vi "insert_block.vi"(8 "direction":enum16{"up", "right", "down", "left"}(ring), 9 "block_type":T1(ring), 10 "position":cluster{"x":u8, "y":u8}, 11 "plate arr":u8[][](array[numeric])) -> (0 "valid?":bool, 3 "return plate":u8[][](array[numeric]))   [LabVIEW 2024]
uses:
  <vilib>/Analysis/coordinate.llb/2D Cartesian Coordinate Rotation (Array).vi
  <vilib>/Analysis/coordinate.llb/2D Cartesian Coordinate Rotation (Scalar).vi
  <vilib>/Analysis/NI_AALPro.lvlib
panel:
  out "熬簿":cluster{"x out":dbl, "y out":dbl}
  # "const table for plaing blocks"
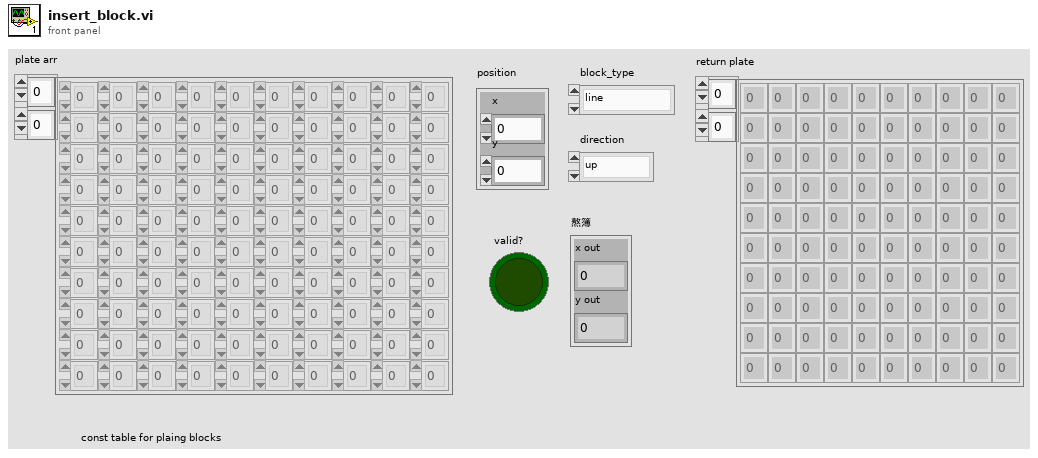
[diagram p1: front panel]
types:
  T1 = enum16{"line", "block", "T", "L", "rev_L", "undefined"}
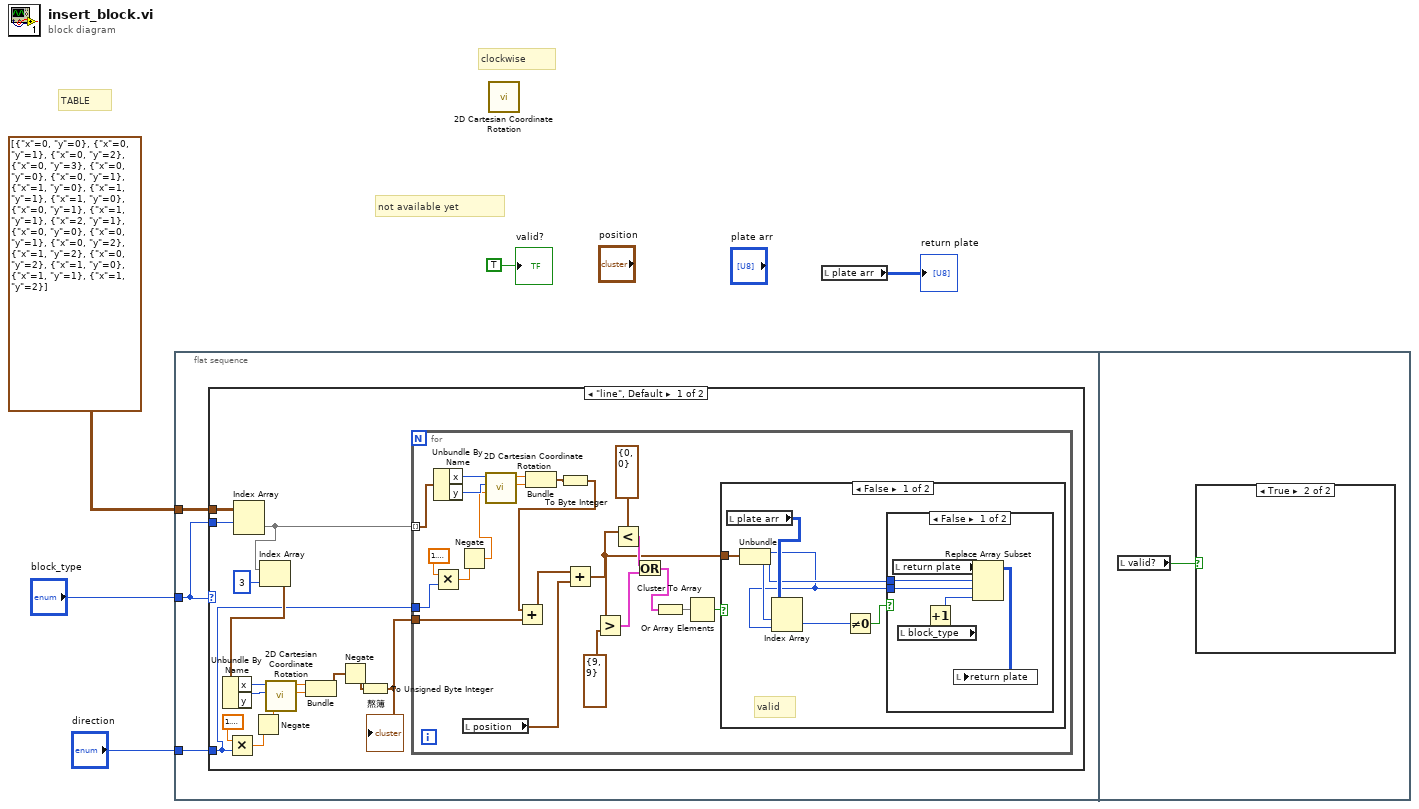
[diagram p0: block diagram]
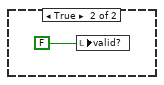
[diagram p2: hidden frame]
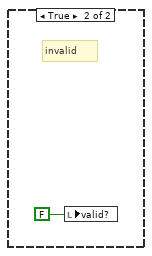
[diagram p3: hidden frame]
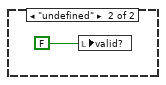
[diagram p4: hidden frame]
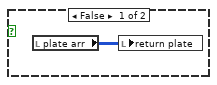
[diagram p5: hidden frame]
diagram:
  # "clockwise"
  # "TABLE"
  # "not available yet"
  n1 = flat-sequence {
    tunnel: cluster{"x":u8, "y":u8}[][] [[{"x"=0, "y"=0}, {"x"=0, "y"=1}, {"x"=0, "y"=2}, {"x"=0, "y"=3}], [{"x"=0, "y"=0}, {"x"=0, "y"=1}, {"x"=1, "y"=0}, {"x"=1, "y"=1}], [{"x"=1, "y"=0}, {"x"=0, "y"=1}, {"x"=1, "y"=1}, {"x"=2, "y"=1}], [{"x"=0, "y"=0}, {"x"=0, "y"=1}, {"x"=0, "y"=2}, {"x"=1, "y"=2}], [{"x"=0, "y"=2}, {"x"=1, "y"=0}, {"x"=1, "y"=1}, {"x"=1, "y"=2}]] ("TABLE") -> [w8]
    tunnel: "block_type" -> [w7]
    tunnel: "direction" -> [w6]
    frame #0 {
      n2 = case shown="\"line\", Default" w7 {
        tunnel: w8 -> [w24 _]
        tunnel: w7 -> [w23 _]
        tunnel: w6 -> [w11 _]
        frame "line", Default {
          n3 = Multiply(x=1.5707963267948966, y=w11) -> (x*y=w17:dbl)
          n4 = Index Array(array=w24, index (row)=w23) -> (element=w22:cluster{"x":u8, "y":u8}[])  [unwired: 1 in]
          n5 = Negate(x=w17) -> (-x=w13:dbl)
          n6 = Index Array(array=w22, index=3) -> (element=w20:cluster{"x":u8, "y":u8})
          n7 = Unbundle By Name(w20) -> ("x"=w19:u8, "y"=w18:u8)
          n8 = call-poly <vilib>:"2D Cartesian Coordinate Rotation.vi"("theta"=w13, "y"=w18, "x"=w19) -> ("y out"=w14:dbl, "x out"=w15:dbl)  [unwired: 6 in, 1 out]
          n9 = Bundle("x out"=w15, "y out"=w14) -> (w10:cluster{"x out":dbl, "y out":dbl})  [unwired: 1 in]
          n10 = Negate(x=w10) -> (-x=w9:cluster{"x out":dbl, "y out":dbl})
          n11 = To Unsigned Byte Integer(number=w9) -> (unsigned 8bit integer=w12:cluster{"x out":u8, "y out":u8})
          "熬簿" <- w12
          n12 = for {
            tunnel: w22 -> [w30] mode=indexing
            tunnel: w12 -> [w31]
            tunnel: w11 -> [w26]
            n13 = Multiply(x=1.5707963267948966, y=w26) -> (x*y=w29:dbl)
            n14 = Unbundle By Name(w30) -> ("x"=w37:u8, "y"=w34:u8)
            n15 = Negate(x=w29) -> (-x=w27:dbl)
            n16 = local read "position"() -> (w32:cluster{"x":u8, "y":u8})
            n17 = call-poly <vilib>:"2D Cartesian Coordinate Rotation.vi"("theta"=w27, "y"=w34, "x"=w37) -> ("y out"=w33:dbl, "x out"=w36:dbl)  [unwired: 6 in, 1 out]
            n18 = Bundle("x out"=w36, "y out"=w33) -> (w35:cluster{"x out":dbl, "y out":dbl})  [unwired: 1 in]
            n19 = To Byte Integer(number=w35) -> (8bit integer=w25:cluster{"x out":i8, "y out":i8})
            n20 = Add(x=w25, y=w31) -> (x+y=w38:cluster{"x out":u8, "y out":u8})
            n21 = Add(x=w38, y=w32) -> (x+y=w39:cluster{u8, u8})
            n22 = Greater?(x=w39, y=cluster{"x":u8, "y":u8} {"x"=9, "y"=9}) -> (0:w43:cluster{bool, bool})
            n23 = Less?(x=w39, y=cluster{"x":u8, "y":u8} {"x"=0, "y"=0}) -> (x < y?=w44:cluster{bool, bool})
            n24 = Or(x=w44, y=w43) -> (x .or. y?=w42:cluster{bool, bool})
            n25 = Cluster To Array(cluster=w42) -> (array=w41:bool[])
            n26 = Or Array Elements(Boolean array=w41) -> (logical OR=w40:bool)
            n27 = case shown="False" w40 {
              tunnel: w39 -> [w52 _]
              frame False {
                # "valid"
                n28 = local read "plate arr"() -> (w51:u8[][])
                n29 = Unbundle(w52) -> (w47:u8, w48:u8)
                n30 = Index Array(array=w51, index (row)=w48, index (col)=w47) -> (element=w50:u8)
                n31 = Not Equal To 0?(x=w50) -> (x != 0?=w49:bool)
                n32 = case shown="False" w49 {
                  tunnel: w48 -> [w57 _]
                  tunnel: w47 -> [w56 _]
                  frame False {
                    n33 = local read "return plate"() -> (w58:u8[][])
                    n34 = local read "block_type"() -> (w54:T1)
                    n35 = Increment(x=w54) -> (x+1=w53:T1)
                    n36 = Replace Array Subset(array=w58, new element=w53, index (row)=w57, index (col)=w56) -> (w55:u8[][])
                    n37 = local write "return plate"(w55) -> ()
                  }
                  frame True {
                    n38 = local write "valid?"(FALSE) -> ()
                  }
                }
              }
              frame True {
                # "invalid"
                n39 = local write "valid?"(FALSE) -> ()
              }
            }
          }
        }
        frame "undefined" {
          n40 = local write "valid?"(FALSE) -> ()
        }
      }
    }
    frame #1 {
      n41 = local read "valid?"() -> (w62:bool)
      n42 = case shown="True" w62 {
        frame False {
          n43 = local read "plate arr"() -> (w63:u8[][])
          n44 = local write "return plate"(w63) -> ()
        }
        frame True {
        }
      }
    }
  }
  n45 = call-poly <vilib>:"2D Cartesian Coordinate Rotation.vi"() -> ()  [unwired: 9 in, 3 out]
  n46 = local read "plate arr"() -> (→"return plate":u8[][])
  "valid?" <- TRUE
